vi "varXNode_Mutate_8_1_0_1.vi"(8 "error in (no error)":errorcluster, 9 "Replies in":string[](array[string]), 10 "Version":T1, 11 "Old State":variant) -> (0 "error out":errorcluster, 1 "Replies out":string[](array[string]), 2 "Version Out":T1, 3 "New State":variant)   [LabVIEW 2017, in "varXNode.xnode"]
uses:
  <vilib>/variable/varXNode.llb/varXNode.xnode
  <vilib>/XNodeSupport/XNodeVersion.ctl
  <vilib>/XNodeSupport/XNodeUShort.ctl
  <vilib>/variable/varXNode.llb/varXNode_old_8_1_0_1.ctl
  <vilib>/variable/Type Descriptor.ctl
  <vilib>/variable/varXNode.llb/varXNode_old_8_1_0_0.ctl
  <vilib>/XNodeSupport/NI_XNodeSupport.lvlib
  <vilib>/variable/NI_Variable.lvlib
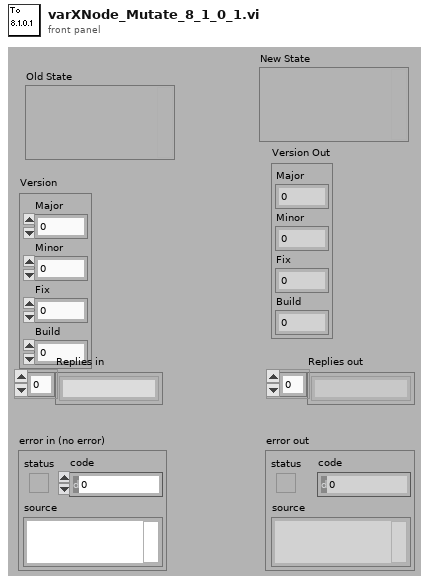
[diagram p1: front panel]
types:
  T1 = typedef "NI_XNodeSupport.lvlib/XNodeVersion.ctl" = cluster{"Major":T2, "Minor":T2, "Fix":T2, "Build":T2}
  T2 = typedef "NI_XNodeSupport.lvlib/XNodeUShort.ctl" = u16
  T3 = typedef "varXNode.xnode/varXNode_old_8_1_0_0.ctl" = cluster{"Write":bool, "ShowTimestamp":bool, "CachedName":string, "CachedTypeDesc":T4, "CachedFeaturePacks":string[], "Custom Rule":string, "ProjectPath":string, "Bad Code":bool, "ContextName":string, "Allow Timestamp":bool}
  T4 = typedef "NI_Variable.lvlib/Type Descriptor.ctl" = cluster{"Variant":variant}
  T5 = typedef "varXNode.xnode/varXNode_old_8_1_0_1.ctl" = cluster{"Write":bool, "ShowTimestamp":bool, "CachedName":string, "CachedTypeDesc":T4, "CachedFeaturePacks":string[], "Custom Rule":string, "ProjectPath":string, "Bad Code":bool, "ContextName":string, "Allow Timestamp":bool, "Generate Code?":bool}
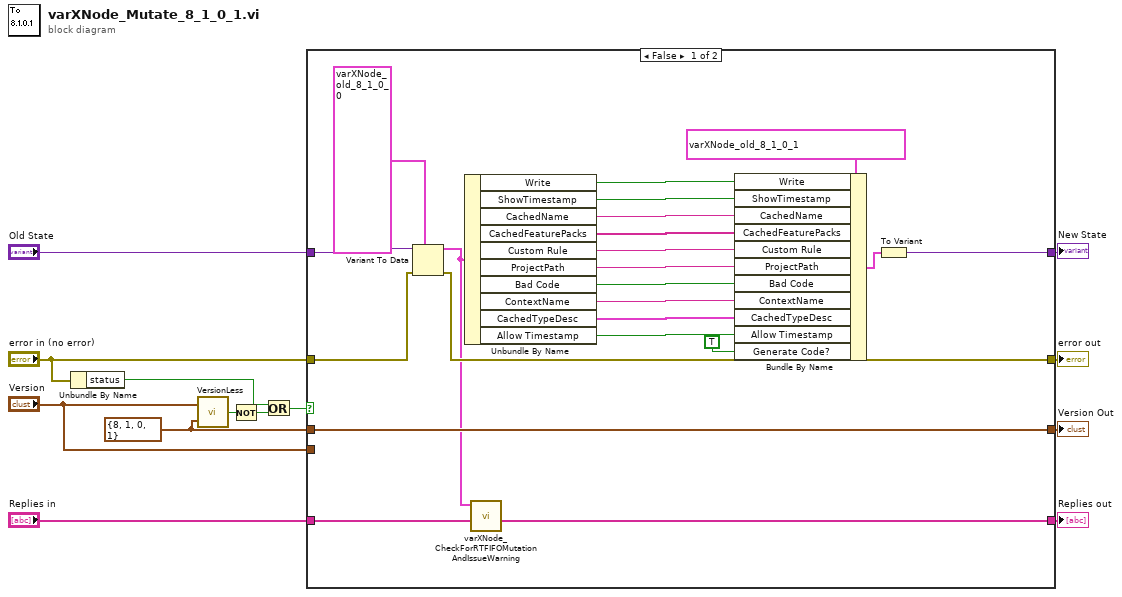
[diagram p0: block diagram]
diagram:
  w12 = T1 {"Major"=8, "Minor"=1, "Fix"=0, "Build"=1} ("y")
  n1 = Unbundle By Name("error in (no error)") -> ("status"=w4:bool)
  n2 = call <vilib>:"VersionLess.vi"("y"=w12, "x"="Version") -> ("x < y?"=w13:bool)
  n3 = Not(x=w13) -> (.not. x?=w3:bool)
  n4 = Or(x=w4, y=w3) -> (x .or. y?=w6:bool)
  n5 = case shown="False" w6 {
    tunnel: w12 -> [w35 _]
    tunnel: [w24 w39] -> w11
    tunnel: "Old State" -> [w34 w39]
    tunnel: [w35 w38] -> w9
    tunnel: "Version" -> [_ w38]
    tunnel: [w19 w37] -> w7
    tunnel: "error in (no error)" -> [w20 w37]
    tunnel: [w17 w36] -> w2
    tunnel: "Replies in" -> [w18 w36]
    frame False {
      n6 = Variant To Data(error in=w20, type=T3 {"Write"=FALSE, "ShowTimestamp"=FALSE, "CachedName"="", "CachedTypeDesc"={"Variant"=variant}, "CachedFeaturePacks"=[], "Custom Rule"="", "ProjectPath"="", "Bad Code"=FALSE, "ContextName"="", "Allow Timestamp"=FALSE} ("State"), Variant=w34) -> (data=w16:T3, error out=w19:errorcluster)
      n7 = Unbundle By Name(w16) -> ("Write"=w32:bool, "ShowTimestamp"=w31:bool, "CachedName"=w30:string, "CachedFeaturePacks"=w29:string[], "Custom Rule"=w28:string, "ProjectPath"=w27:string, "Bad Code"=w26:bool, "ContextName"=w25:string, "CachedTypeDesc"=w21:T4, "Allow Timestamp"=w14:bool)
      n8 = call <vilib>:"varXNode_CheckForRTFIFOMutationAndIssueWarning.vi"("Replies in"=w18, "State"=w16) -> ("Replies out"=w17:string[])  [unwired: 9 in]
      n9 = Bundle By Name(cluster=T5 {"Write"=FALSE, "ShowTimestamp"=FALSE, "CachedName"="", "CachedTypeDesc"={"Variant"=variant}, "CachedFeaturePacks"=[], "Custom Rule"="", "ProjectPath"="", "Bad Code"=FALSE, "ContextName"="", "Allow Timestamp"=FALSE, "Generate Code?"=FALSE} ("State"), "Write"=w32, "ShowTimestamp"=w31, "CachedName"=w30, "CachedFeaturePacks"=w29, "Custom Rule"=w28, "ProjectPath"=w27, "Bad Code"=w26, "ContextName"=w25, "CachedTypeDesc"=w21, "Allow Timestamp"=w14, "Generate Code?"=TRUE) -> (w23:T5)
      n10 = To Variant(anything=w23) -> (Variant=w24:variant)
    }
    frame True {
      # "Either there was an error in,\nor the version is not less than 1.0.0.6.\nPass input values out."
    }
  }
  "New State" <- w11
  "Version Out" <- w9
  "error out" <- w7
  "Replies out" <- w2
